vi "Open.vi"(8 "error in (no error)":errorcluster caption="entrée d'erreur (pas d'erreur)", 11 "Class Relay_Board 16_Relay_R4D3D16 en entrée":refnum<class "Class Relay_Board 8_Relay_N4D8B08.lvclass">) -> (0 "error out":errorcluster caption="sortie d'erreur", 3 "Class Relay_Board 16_Relay_R4D3D16 en sortie":refnum<class "Class Relay_Board 8_Relay_N4D8B08.lvclass">)   [LabVIEW 2020, in "Library Instrument & Equipement.lvlib" / "Library Relay_Board.lvlib" / "Class Relay_Board 8_Relay_N4D8B08.lvclass"]
uses:
  Class Relay_Board 8_Relay_N4D8B08.lvclass
  C:/Users/ngarcin/OneDrive - Altyor/Standard TB/Class/Relay_Board/Relay_Board (Default)/Class Relay_Board (Default).lvclass
  Class Relay_Board 8_Relay_N4D8B08.lvclass/Class Relay_Board 8_Relay_N4D8B08.ctl
  Modbus/Modbus.lvclass
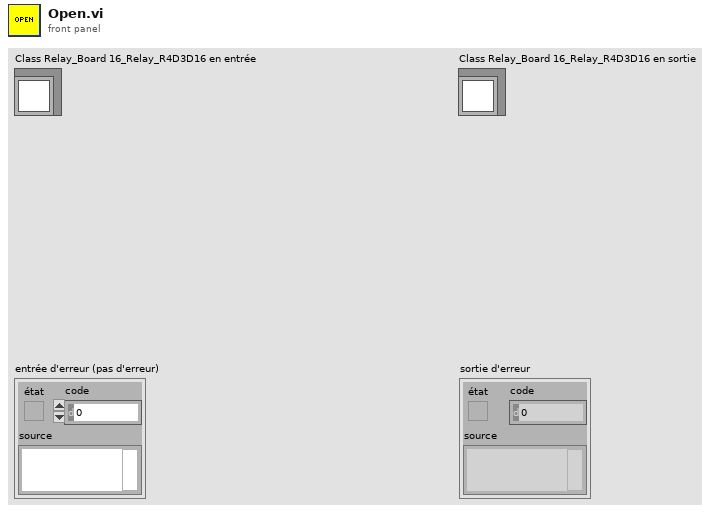
[diagram p1: front panel]
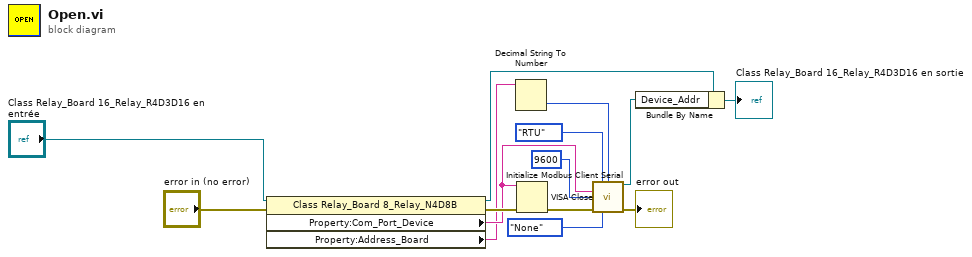
[diagram p0: block diagram]
diagram:
  n1 = property class="Class Relay_Board 8_Relay_N4D8B"(reference="Class Relay_Board 16_Relay_R4D3D16 en entrée", error in="error in (no error)") -> (reference out=w11:refnum<class "Class Relay_Board 8_Relay_N4D8B08.lvclass">, error out=w12:errorcluster, "Property:Com_Port_Device"=w8:string, "Property:Address_Board"=w4:string)
  n2 = Decimal String To Number(string=w4) -> (number=w3:i32)  [unwired: 2 in, 1 out]
  n3 = VISA Close(VISA resource name=w8, error in (no error)=w12) -> (error out=w9:errorcluster)
  n4 = call "Initialize Modbus Client Serial.vi"("protocol (RTU)"=enum16{"RTU", "ASCII", "TCP"}."RTU", "station address (1)"=w3, "port"=w8, "baud rate (9600)"=u32 9600, "error in (no error)"=w9, "parity (even)"=enum16{"None", "Odd", "Even", "Mark", "Space"}."None") -> ("MODBUS Out"=w1:refnum<class "Modbus.lvclass">, "error out"=→"error out":errorcluster)  [unwired: 8 in]
  n5 = Bundle By Name(cluster=w11, "Device_Addr"=w1) -> (→"Class Relay_Board 16_Relay_R4D3D16 en sortie":refnum<class "Class Relay_Board 8_Relay_N4D8B08.lvclass">)
